vi "ntr.log-parse.unit-sample.vi"(10 "log":T1={"Proc Name"="NUTRITION", "ProcPath"="C:\\interface\\procedures\\NUTRITION.prc", "Step Name"="_UNIT_SAMPLE", "Step Function"=enum."UNIT_SAMPLE", "Step Index"=9, "Report"="UNIT=1;EC=2.2 LOW;PH=-33.6 ALARM;ORP=-33.6 ALARM;UNWL_1=1.0 RANGE;UNWT_1=-33.6", "clk"=3807513890.0668745, "error in"={"status"=FALSE, "code"=0, "source"=""}, "Log Message"="", "Proc Module"=""} {"clk" format="%#.3f"}, 11 "status-table-REF":refnum<vi>) -> (3 "ntr.status-table":string[][](table)=[["Range", "High", "Low", "25", "FULL"], ["", "", "", "", ""], ["", "", "", "", ""], ["", "", "", "", ""], ["", "", "", "", ""], ["", "", "", "", ""], ["", "", "", "", ""], ["", "", "", "", ""], ["", "", "", "", ""]])   [LabVIEW 2024]
uses:
  controls/typeEngineLogCluster.ctl
  controls/type.StepFunction.ctl
  controls/typePathSelector.ctl
  <vilib>/Utility/miscctls.llb/LVRowAndColumnTypeDef.ctl
  <vilib>/Utility/error.llb/Clear Errors.vi
  <vilib>/Utility/libraryn.llb/Create Directory Recursive.vi
  <vilib>/Utility/file.llb/Write Delimited Spreadsheet (string).vi
  <vilib>/Utility/file.llb/Read Delimited Spreadsheet (string).vi
panel:
  out "MSG":string[](array[string])
  out "NAMES":string[](array[string])
  out "VALUES":string[](array[string])
  out "filenames":string[](array[string])
  out "SelectedPath":path
  out "row idx":i32
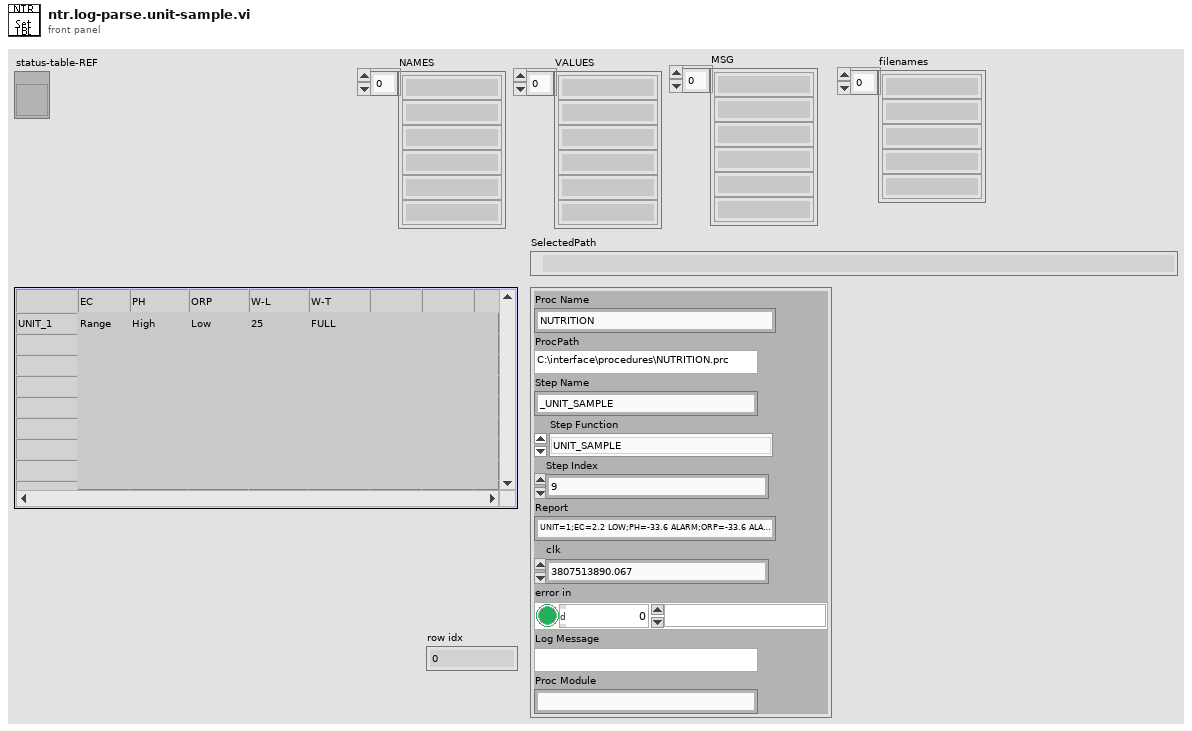
[diagram p1: front panel]
types:
  T1 = typedef "typeEngineLogCluster.ctl" = cluster{"Proc Name":string, "ProcPath":string, "Step Name":string, "Step Function":T2, "Step Index":i32, "Report":string, "clk":dbl, "error in":errorcluster, "Log Message":string, "Proc Module":string}
  T2 = typedef "type.StepFunction.ctl" = enum16{"__NO-OP", "_DELAY_LOAD", "_DELAY_COMPARE", "_JUMP", "_COMPLETE", "_COMPARE", "_LOG_MESSAGE", "_LOG_LAST_REPORT", "_SCHEDULE", "_SCHED_DAILY", "CLK_COMPARE", "PROC_START", "PROC_STOP", "PROC_LOAD", "PROC_COMPLETION_CHECK", "PROC_COMPLETION_LOAD", "_IO_READ", "_IO_READ_MANY", "_IO_WRITE", "_IO_WRITE_BY_REG", "_IO_GET_OUTPUT", "_OCS_CHECK", "_OCS_RECORD", "_GET_RH", "_GET_ACC_UV", "_GET_WD", "_GET_WS", "_REC_DELETE", "_REC_MOVE", "_REC_COPY", "_IRR_CHECK", "UNIT_CHECK", "UNIT_SAMPLE", "UNIT_DOSE"}
  T3 = typedef "LVRowAndColumnTypeDef.ctl" = cluster{"Row":i32, "Column":i32}
  T4 = typedef "typePathSelector.ctl" = enum16{"DIR_PROCS", "DIR_CONFIG", "DIR_TEMPLATE", "DIR_IO_FILE", "DIR_RECORD", "DIR_LOG", "DIR_RUNTIME", "DIR_PRESET", "DIR_INI"}
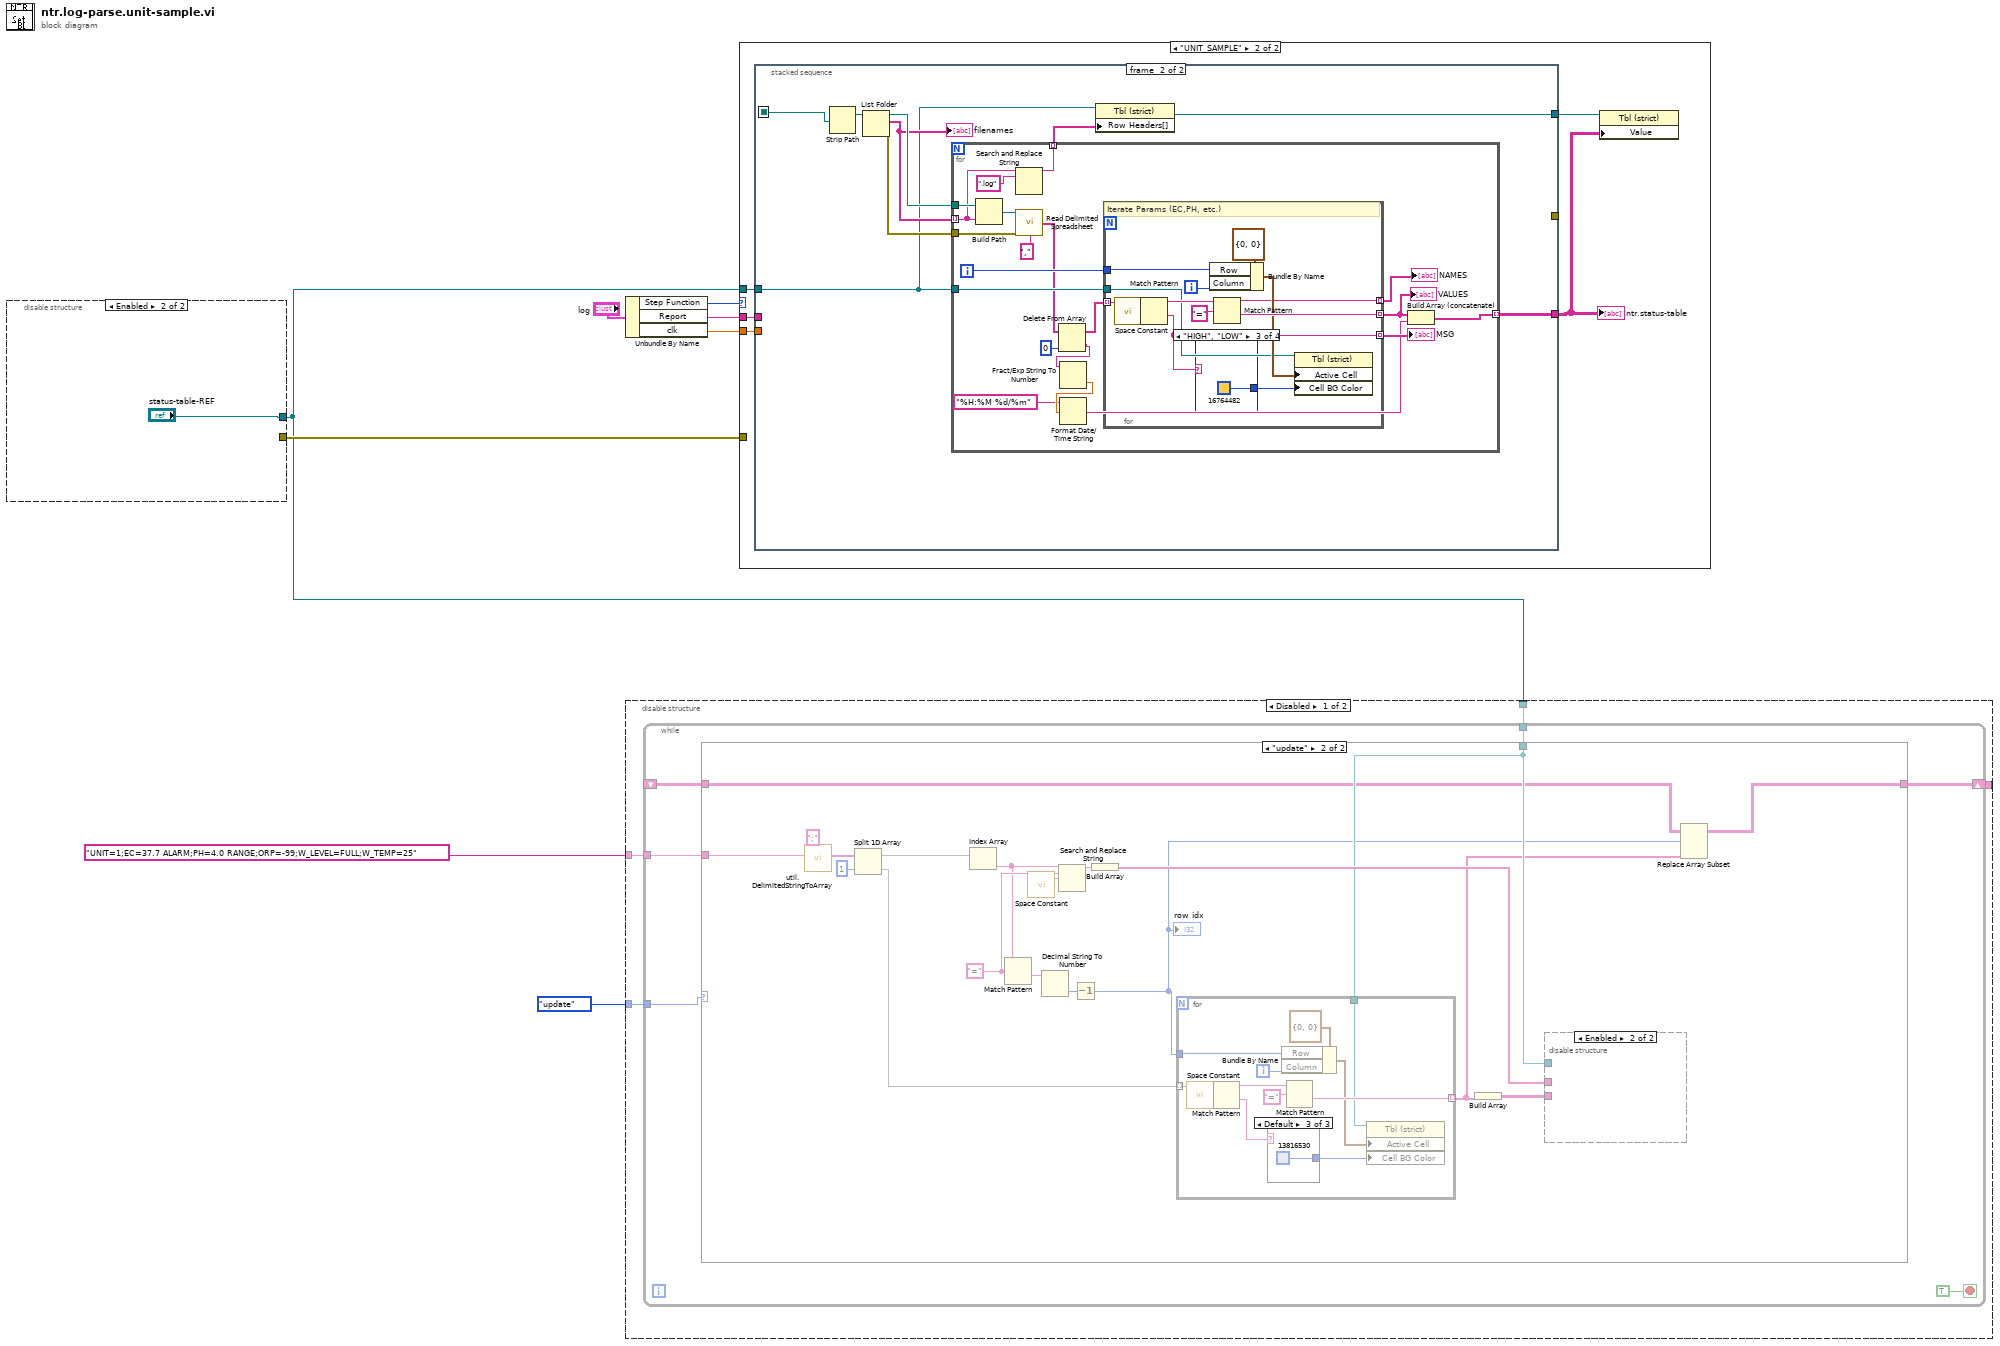
[diagram p0: block diagram]
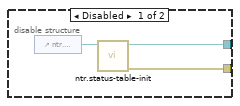
[diagram p2: hidden frame]
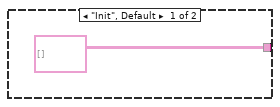
[diagram p3: hidden frame]
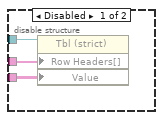
[diagram p4: hidden frame]
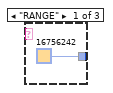
[diagram p5: hidden frame]
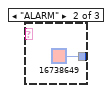
[diagram p6: hidden frame]
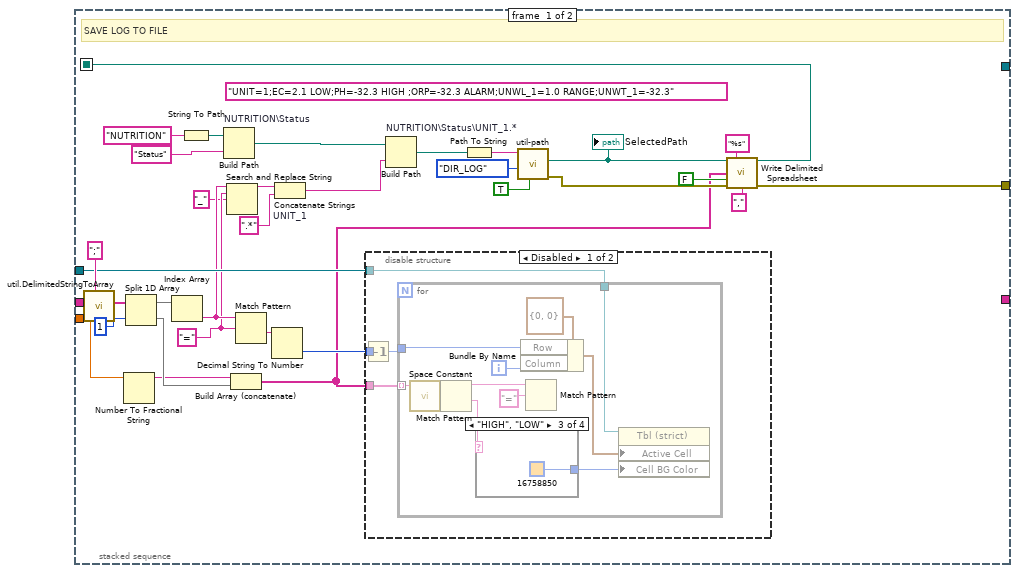
[diagram p9: hidden frame]
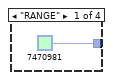
[diagram p10: hidden frame]
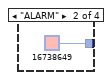
[diagram p11: hidden frame]
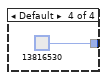
[diagram p12: hidden frame]
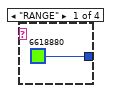
[diagram p14: hidden frame]
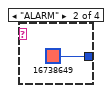
[diagram p15: hidden frame]
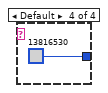
[diagram p16: hidden frame]
diagram:
  n1 = disable-structure shown="Enabled" {
    disable-tunnel: [w11 _] -> w3
    disable-tunnel: [w10 "status-table-REF"] -> w2
    frame Disabled {
      n2 = control-ref of="ntr.status-table"() -> (w9:refnum<vi>)
      n3 = call "ntr.status-table-init.vi"("Table in"=w9) -> ("error out"=w11:errorcluster, "Table out"=w10:refnum<vi>)  [unwired: 9 in]
    }
    frame Enabled {
    }
  }
  n4 = disable-structure shown="Disabled" {
    disable-tunnel: "UNIT=1;EC=37.7 ALARM;PH=4.0 RANGE;ORP=-99;W_LEVEL=FULL;W_TEMP=25" ("String") -> [w16 _]
    disable-tunnel: enum16{"Init", "update"}."update" -> [w15 _]
    disable-tunnel: [w14 _] -> _
    disable-tunnel: w2 -> [w13 _]
    frame Disabled {
      n5 = while {
        tunnel: w16 -> [w22]
        tunnel: w13 -> [w21]
        shift-right: [w20] -> w14
        shift-left: _ -> [w19]
        tunnel: w15 -> [w18]
        stop <- TRUE stop-if-true
        n6 = case shown="\"update\"" w18 {
          tunnel: w22 -> [_ w42]
          tunnel: w21 -> [_ w29]
          tunnel: [string[][] [] ("ntr.status-table") w25] -> w20
          tunnel: w19 -> [_ w24]
          frame "Init", Default {
          }
          frame "update" {
            w37 = "=" ("regular expression")
            n7 = call "util.DelimitedStringToArray.vi"("delimiter (,)"=";", "delimitaed string"=w42) -> ("array out"=w40:string[])  [unwired: 9 in]
            n8 = Split 1D Array(array=w40, index=1) -> (first subarray=w33:string[], second subarray=w30:string[])
            n9 = Index Array(array=w33) -> (element=w32:string)  [unwired: 1 in]
            n10 = Match Pattern(string=w32, regular expression=w37) -> (after substring=w39:string)  [unwired: 1 in, 3 out]
            n11 = call <vilib>:"Space Constant.vi"() -> ("String"=w36:string)
            n12 = Decimal String To Number(string=w39) -> (number=w38:i32)  [unwired: 2 in, 1 out]
            n13 = Search and Replace String(input string=w32, search string=w37, replace string=w36) -> (result string=w35:string)  [unwired: 5 in, 3 out]
            n14 = Decrement(x=w38) -> (x-1=w27:i32)
            "row idx" <- w27
            n15 = Build Array(w35) -> (w34:string[])
            n16 = for {
              tunnel: w30 -> [w57] mode=indexing
              tunnel: [w53] -> w26 mode=indexing
              tunnel: w27 -> [w51]
              tunnel: w29 -> [w49]
              i -> [w50]
              n17 = call <vilib>:"Space Constant.vi"() -> ("String"=w56:string)
              n18 = Match Pattern(string=w57, regular expression=w56) -> (before substring=w54:string, after substring=w52:string)  [unwired: 1 in, 2 out]
              n19 = case shown="Default" w52 {
                tunnel: [u32 16756242 u32 16738649 u32 13816530] -> w47
                frame "RANGE" {
                }
                frame "ALARM" {
                }
                frame Default {
                }
              }
              n20 = Bundle By Name(cluster=T3 {"Row"=0, "Column"=0} ("Active Cell:Active Cell"), "Row"=w51, "Column"=w50) -> (w48:T3)
              n21 = Match Pattern(string=w54, regular expression="=") -> (after substring=w53:string)  [unwired: 1 in, 3 out]
              n22 = property class="Tbl (strict)"(reference=w49, "Active Cell"=w48, "Cell BG Color"=w47) -> ()  [unwired: 1 in, 2 out]
            }
            n23 = Build Array(w26) -> (w28:string[][])
            n24 = disable-structure shown="Enabled" {
              disable-tunnel: w34 -> [w45 _]
              disable-tunnel: w29 -> [w44 _]
              disable-tunnel: w28 -> [w43 _]
              frame Disabled {
                n25 = property class="Tbl (strict)"(reference=w44, "Row Headers[]"=w45, "Value"=w43) -> ()  [unwired: 1 in, 2 out]
              }
              frame Enabled {
              }
            }
            n26 = Replace Array Subset(array=w24, new element=w26, index (row)=w27) -> (w25:string[][])  [unwired: 1 in]
          }
        }
      }
    }
    frame Enabled {
    }
  }
  n27 = Unbundle By Name("log") -> ("Step Function"=w5:T2, "Report"=w4:string, "clk"=w1:dbl)
  n28 = case shown="\"UNIT_SAMPLE\"" w5 {
    tunnel: w4 -> [_ w65]
    tunnel: w2 -> [_ w64]
    tunnel: w3 -> [_ _]
    tunnel: w1 -> [_ w61]
    frame Default {
    }
    frame "UNIT_SAMPLE" {
      n29 = stacked-sequence {
        seq-local: [w71 _] -> [_ w126]
        tunnel: w65 -> [w96 _]
        tunnel: w64 -> [w91 w120]
        tunnel: [w69 _] -> _
        tunnel: [_ w121] -> w62
        tunnel: [_ w118] -> w63
        tunnel: w61 -> [w67 _]
        frame #0 {
          w89 = "=" ("regular expression")
          (unwired) "UNIT=1;EC=2.1 LOW;PH=-32.3 HIGH ;ORP=-32.3 ALARM;UNWL_1=1.0 RANGE;UNWT_1=-32.3" ("String")
          # "SAVE LOG TO FILE"
          n30 = call "util.DelimitedStringToArray.vi"("delimiter (,)"=";", "delimitaed string"=w96) -> ("array out"=w98:string[])  [unwired: 9 in]
          n31 = Number To Fractional String(number=w67) -> (F-format string=w66:string)  [unwired: 3 in]
          n32 = Split 1D Array(array=w98, index=1) -> (first subarray=w94:string[], second subarray=w76:string[])
          n33 = Index Array(array=w94) -> (element=w90:string)  [unwired: 1 in]
          n34 = String To Path(string="NUTRITION") -> (path=w87:path)
          n35 = Build Path "NUTRITION\\Status"(base path=w87, name or relative path="Status" ("string")) -> (appended path=w82:path)
          n36 = Search and Replace String(input string=w90, search string=w89, replace string="_" ("replace string (\"\")")) -> (result string=w85:string)  [unwired: 5 in, 3 out]
          n37 = Build Array (concatenate)(w66, w76) -> (w68:string[])
          n38 = Match Pattern(string=w90, regular expression=w89) -> (after substring=w92:string)  [unwired: 1 in, 3 out]
          n39 = Decimal String To Number(string=w92) -> (number=w93:i32)  [unwired: 2 in, 1 out]
          n40 = Concatenate Strings "UNIT_1"(w85, ".*" ("string")) -> (w81:string)
          n41 = disable-structure shown="Disabled" {
            disable-tunnel: w93 -> [w102 _]
            disable-tunnel: w91 -> [w100 _]
            disable-tunnel: w68 -> [w99 _]
            frame Disabled {
              n42 = Decrement(x=w102) -> (x-1=w101:i32)
              n43 = for {
                tunnel: w99 -> [w113] mode=indexing
                tunnel: w101 -> [w108]
                tunnel: w100 -> [w106]
                i -> [w107]
                n44 = call <vilib>:"Space Constant.vi"() -> ("String"=w112:string)
                n45 = Match Pattern(string=w113, regular expression=w112) -> (before substring=w110:string, after substring=w109:string)  [unwired: 1 in, 2 out]
                n46 = case shown="\"HIGH\", \"LOW\"" w109 {
                  tunnel: [u32 7470981 u32 16738649 u32 16758850 u32 13816530] -> w104
                  frame "RANGE" {
                  }
                  frame "ALARM" {
                  }
                  frame "HIGH", "LOW" {
                  }
                  frame Default {
                  }
                }
                n47 = Bundle By Name(cluster=T3 {"Row"=0, "Column"=0} ("Active Cell:Active Cell"), "Row"=w108, "Column"=w107) -> (w105:T3)
                n48 = Match Pattern(string=w110, regular expression="=") -> ()  [unwired: 1 in, 4 out]
                n49 = property class="Tbl (strict)"(reference=w106, "Active Cell"=w105, "Cell BG Color"=w104) -> ()  [unwired: 1 in, 2 out]
              }
            }
            frame Enabled {
            }
          }
          n50 = Build Path "NUTRITION\\Status\\UNIT_1.*"(base path=w82, name or relative path=w81) -> (appended path=w80:path)
          n51 = Path To String(path=w80) -> (string=w79:string)
          n52 = call "util-path.vi"("Create Folders?(F)"=TRUE, "Selected Folder (PROCS)"=typePathSelector."DIR_LOG" ("Selected Folder (PROCEDURE_DIR)"), "append path (ie. folder\\filename.*)"=w79) -> ("error out"=w70:errorcluster, "SelectedPath"=w73:path)  [unwired: 4 in, 3 out]
          "SelectedPath" <- w73
          n53 = call-poly <vilib>:"Write Delimited Spreadsheet.vi"("file path (dialog if empty)"=w73, "format (%s)"="%s", "1D data"=w68, "append to file? (new file:F)"=FALSE, "error in (no error)"=w70, "delimiter (\\t)"="," ("delimiter (\\t)")) -> ("new file path (Not A Path if cancelled)"=w71:path, "error out"=w69:errorcluster)  [unwired: 8 in]
        }
        frame #1 {
          n54 = Strip Path(path=w126) -> (stripped path=w125:path)  [unwired: 1 out]
          n55 = List Folder(path=w125) -> (path out=w124:path, filenames=w123:string[], error out=w122:errorcluster)  [unwired: 3 in, 1 out]
          "filenames" <- w123
          n56 = for {
            tunnel: w124 -> [w146]
            tunnel: w123 -> [w137] mode=indexing
            tunnel: w122 -> [w143]
            tunnel: w120 -> [w141]
            tunnel: [w131] -> w121 mode=indexing
            tunnel: [w135] -> w119 mode=indexing
            i -> [w142]
            n57 = Build Path(base path=w146, name or relative path=w137) -> (appended path=w145:path)
            n58 = Search and Replace String(input string=w137, search string=".log") -> (result string=w135:string)  [unwired: 6 in, 3 out]
            n59 = call-poly <vilib>:"Read Delimited Spreadsheet.vi"("file path (dialog if empty)"=w145, "error in (no error)"=w143, "delimiter (\\t)"="," ("delimiter (\\t)")) -> ("first row"=w134:string[])  [unwired: 7 in, 5 out]
            n60 = Delete From Array(array=w134, index=0) -> (deleted portion=w130:string, array with subset deleted=w133:string[])  [unwired: 1 in]
            n61 = Fract/Exp String To Number(string=w130) -> (number=w129:dbl)  [unwired: 3 in, 1 out]
            n62 = Format Date/Time String(time format string (%c)="%H:%M %d/%m", seconds (now)=w129) -> (date/time string=w128:string)  [unwired: 1 in]
            n63 = for {
              tunnel: [w156] -> w139 mode=indexing
              tunnel: w142 -> [w155]
              tunnel: [w150] -> w140 mode=indexing
              tunnel: w141 -> [w149]
              tunnel: w133 -> [w148] mode=indexing
              tunnel: [w147] -> w138 mode=indexing
              i -> [w154]
              # "Iterate Params (EC,PH, etc.)"
              n64 = call <vilib>:"Space Constant.vi"() -> ("String"=w159:string)
              n65 = Match Pattern(string=w148, regular expression=w159) -> (before substring=w157:string, after substring=w147:string)  [unwired: 1 in, 2 out]
              n66 = case shown="\"HIGH\", \"LOW\"" w147 {
                tunnel: [u32 6618880 u32 16738649 u32 16764482 u32 13816530] -> w152
                frame "RANGE" {
                }
                frame "ALARM" {
                }
                frame "HIGH", "LOW" {
                }
                frame Default {
                }
              }
              n67 = Bundle By Name(cluster=T3 {"Row"=0, "Column"=0} ("Active Cell:Active Cell"), "Row"=w155, "Column"=w154) -> (w153:T3)
              n68 = Match Pattern(string=w157, regular expression="=") -> (before substring=w150:string, after substring=w156:string)  [unwired: 1 in, 2 out]
              n69 = property class="Tbl (strict)"(reference=w149, "Active Cell"=w153, "Cell BG Color"=w152) -> ()  [unwired: 1 in, 2 out]
            }
            "VALUES" <- w139
            "NAMES" <- w140
            "MSG" <- w138
            n70 = Build Array (concatenate)(w139, w128) -> (w131:string[])
          }
          n71 = property class="Tbl (strict)"(reference=w120, "Row Headers[]"=w119) -> (reference out=w118:refnum<vi>)  [unwired: 1 in, 1 out]
        }
      }
      "ntr.status-table" <- w62
      n72 = property class="Tbl (strict)"(reference=w63, "Value"=w62) -> ()  [unwired: 1 in, 2 out]
    }
  }
